vi "Autonomous Independent.vi"   [LabVIEW 2020]
doc: "This VI is called when autonomous begins, and will automatically be terminated when autonomous ends. You can carry out timed or sensor driven robot movement independently without needing to return to the caller."
uses:
  <vilib>/Rock Robotics/WPI/ThirdParty/Phoenix-LabVIEW/Motor Controller/Controls/CTRE_Phoenix_MotorControl_ControlMode.ctl
  <vilib>/Rock Robotics/WPI/Solenoid/WPI_SolenoidValue.ctl
  <vilib>/Rock Robotics/WPI/Utilities/WPI_GetSetVariantRefNum.vi
  <vilib>/Rock Robotics/Network Tables/NT Read String.vi
  <vilib>/Rock Robotics/Network Tables/NT Write Numeric Array.vi
  <vilib>/Rock Robotics/WPI/Solenoid/WPI_SolenoidSetEnum.vi
panel:
  # "Be sure to right-click and choose Data Operations>>Make Current Value default if you want to save the array values with the VI"
types:
  T1 = typedef "WPI_JoystickDevRef.ctl" = cluster{"Device":T2}
  T2 = typedef "WPI_JoystickDeviceEnum.ctl" = enum16{"USB 0", "USB 1", "USB 2", "USB 3", "USB 4", "USB 5"}
  T3 = typedef "WPI_MotorControlDeviceRef.ctl" = cluster{"DeviceStatus":errorcluster, "Type":T4, "PWM":cluster{"PWM Channel":T5, "DeadBand":T6}, "CAN":cluster{"Device Number":u8, "SetOutput VI Ref":variant, "GetOutput VI Ref":variant, "Enable VI Ref":variant, "Disable VI Ref":variant, "Data":variant}, "Invert":bool, "DIO PWM":cluster{"PWM \"Enable\" Channel":T5, "DIOChannel":T7, "PWM Rate":dbl}}
  T4 = typedef "WPI_MotorControlType.ctl" = enum16{"PWM", "CAN", "DIO PWM"}
  T5 = typedef "FPGA_DIOPWMChannel.ctl" = enum8{"PWM 0", "PWM 1", "PWM 2", "PWM 3", "PWM 4", "PWM 5", "PWM 6", "PWM 7", "PWM 8", "PWM 9", "PWM MXP 0", "PWM MXP 1", "PWM MXP 2", "PWM MXP 3", "PWM MXP 4", "PWM MXP 5", "PWM MXP 6", "PWM MXP 7", "PWM MXP 8", "PWM MXP 9", "Invalid"}
  T6 = typedef "WPI_PWMDeadband.ctl" = cluster{"Name":string, "maxPositivePwm":i32, "minPositivePwm":i32, "centerPwm":i32, "maxNegativePwm":i32, "minNegativePwm":i32, "angularRange":u16}
  T7 = typedef "FPGA_DIOChannel.ctl" = enum8{"DIO 0", "DIO 1", "DIO 2", "DIO 3", "DIO 4", "DIO 5", "DIO 6", "DIO 7", "DIO 8", "DIO 9", "DIO MXP 0", "DIO MXP 1", "DIO MXP 2", "DIO MXP 3", "DIO MXP 4", "DIO MXP 5", "DIO MXP 6", "DIO MXP 7", "DIO MXP 8", "DIO MXP 9", "DIO MXP 10", "DIO MXP 11", "DIO MXP 12", "DIO MXP 13", "DIO MXP 14", "DIO MXP 15", "SPI Port CS1", "SPI Port CS2", "SPI Port CS3", "SPI Port MISO", "SPI Port MOSI", "Invalid"}
  T8 = typedef "WPI_RobotDriveDevRef.ctl" = cluster{"DevStatus":errorcluster, "Motors[]":T3[], "Square Inputs":bool, "Max Output":dbl}
  T9 = typedef "WPI_SolenoidDevRef.ctl" = cluster{"DevStatus":errorcluster, "Pneumatics Control Module":u8, "Forward Solenoid Channel":T10, "Reverse Solenoid Channel":T10}
  T10 = typedef "WPI_SolenoidChannel.ctl" = enum8{"Solenoid 0", "Solenoid 1", "Solenoid 2", "Solenoid 3", "Solenoid 4", "Solenoid 5", "Solenoid 6", "Solenoid 7", "Solenoid 8", "Solenoid 9", "Solenoid 10", "Solenoid 11", "Solenoid 12", "Solenoid 13", "Solenoid 14", "Solenoid 15", "Invalid"}
  T11 = typedef "WPI_DigitalInputDevRef.ctl" = cluster{"DevStatus":errorcluster, "DIO Channel":T7}
  T12 = typedef "WPI_SolenoidValue.ctl" = enum16{"Off", "On", "Forward", "Reverse"}
  T13 = typedef "CTRE_Phoenix_MotorControl_ControlMode.ctl" = u16
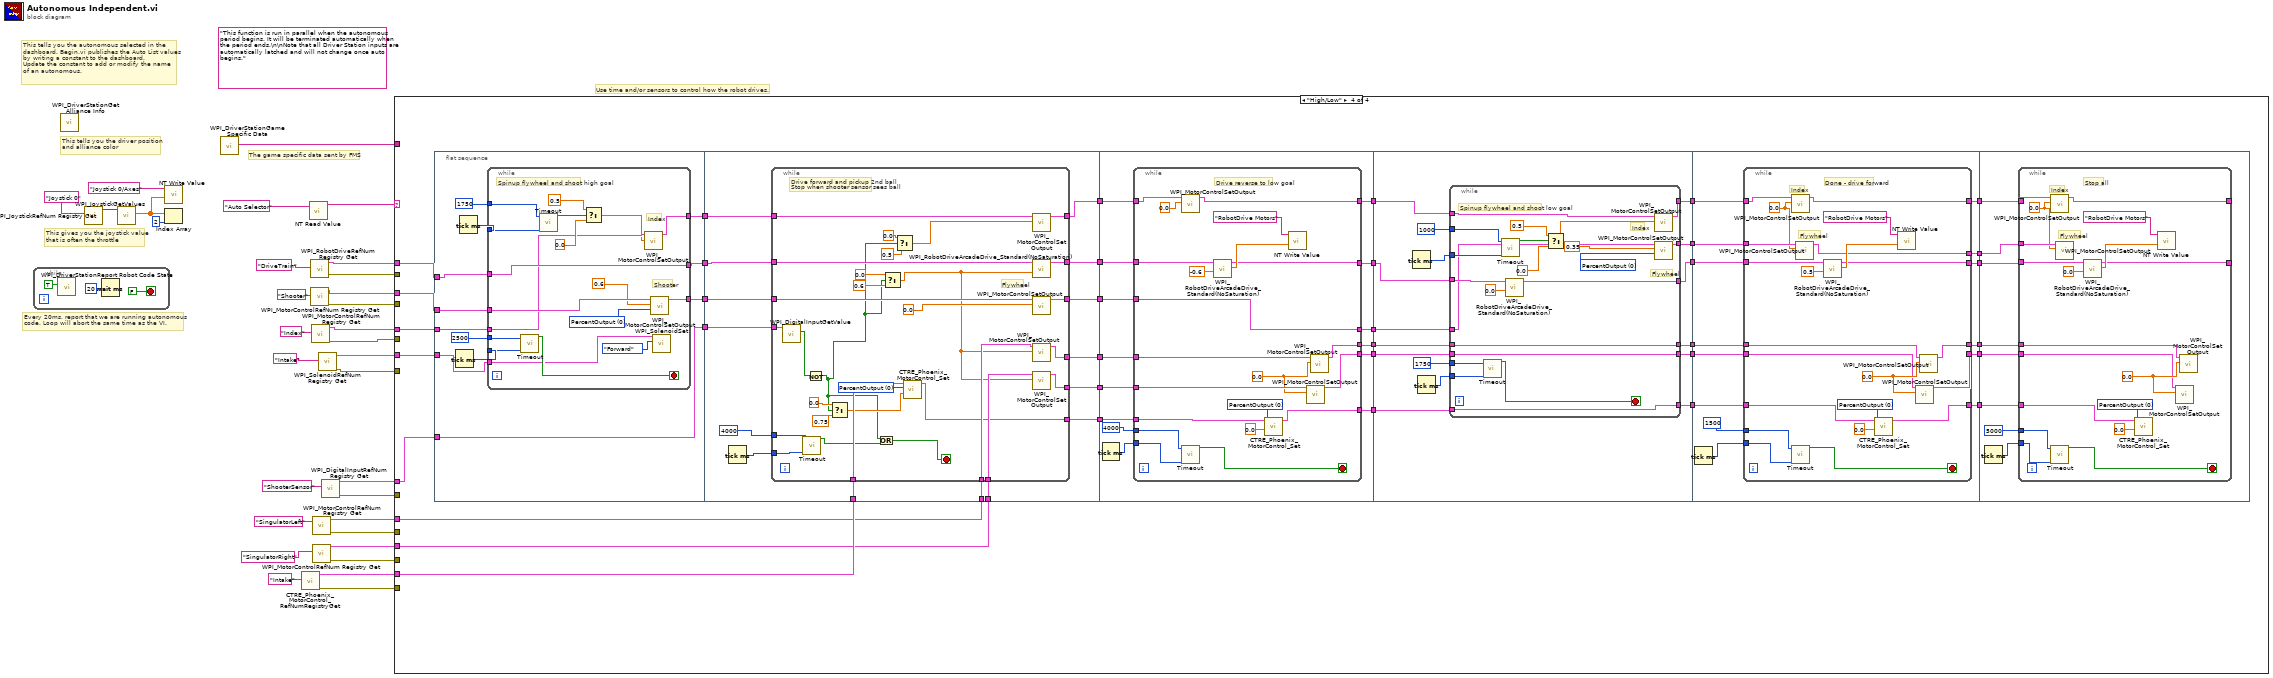
[diagram p0: block diagram]
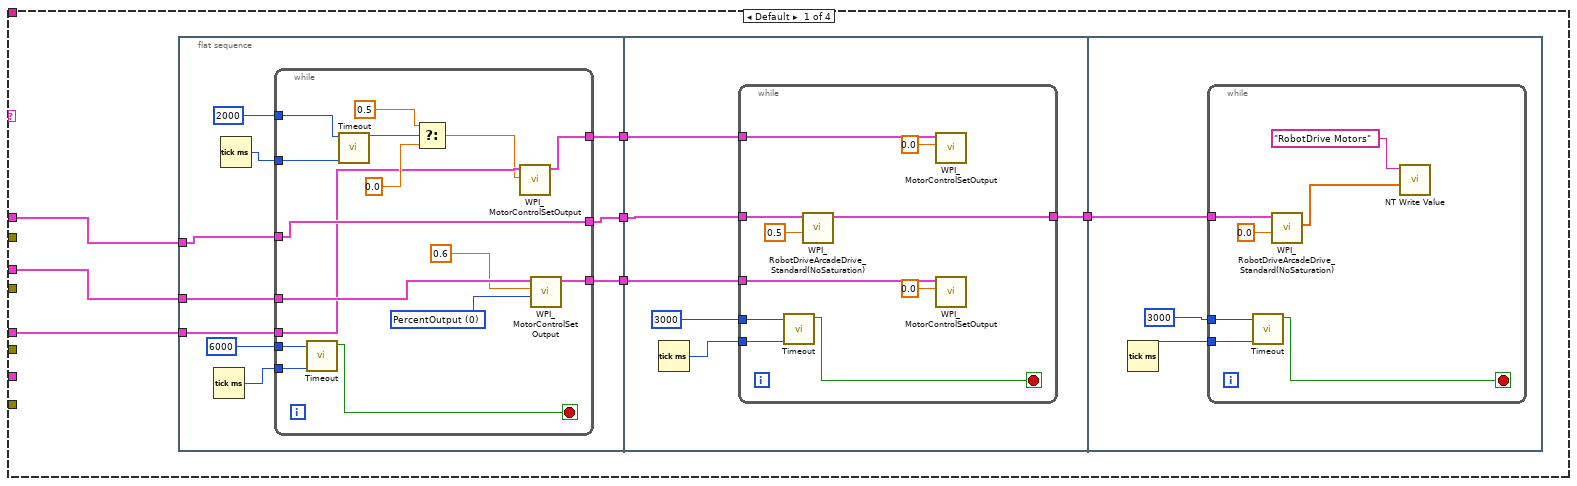
[diagram p2: hidden frame]
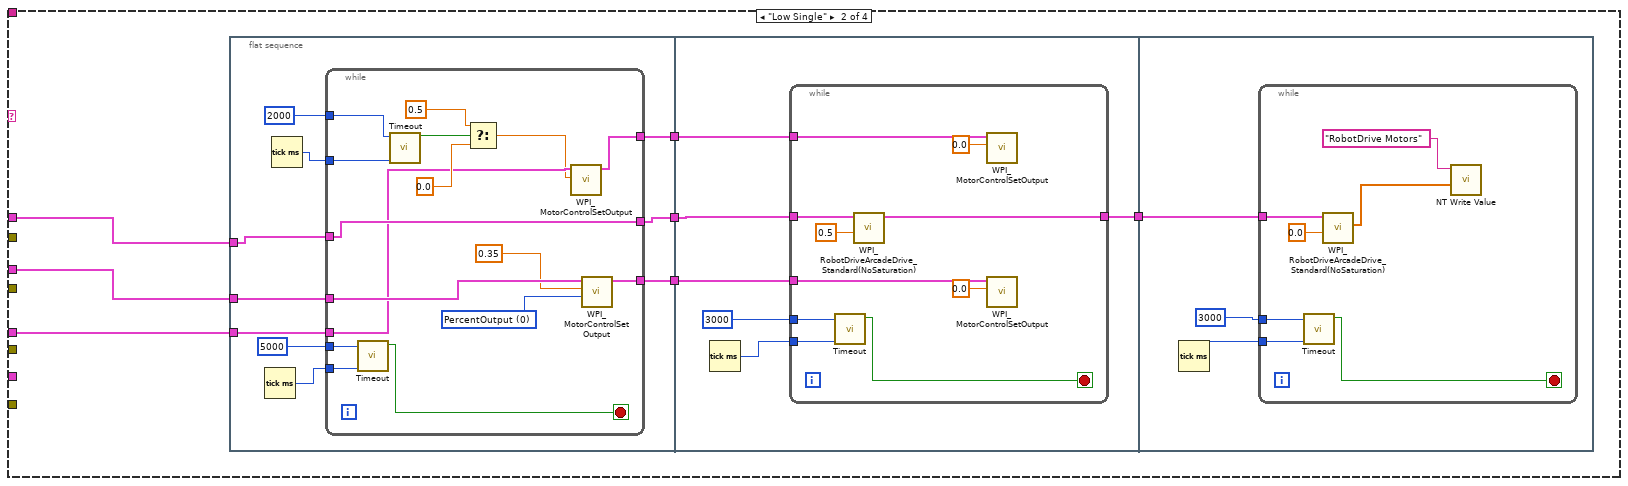
[diagram p3: hidden frame]
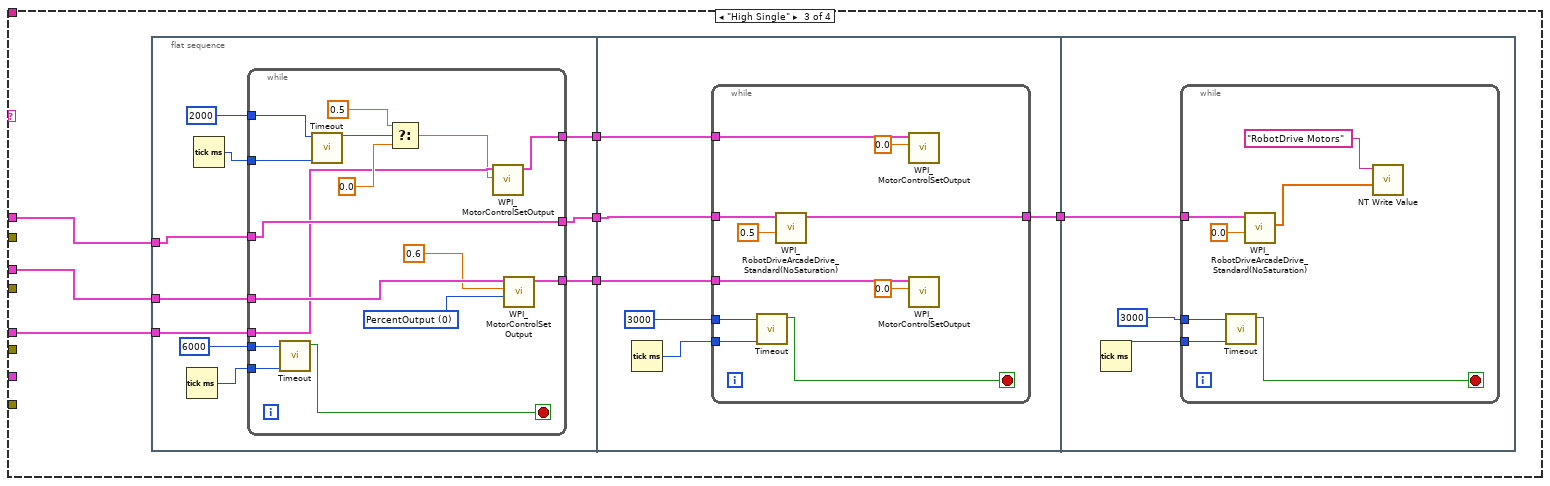
[diagram p4: hidden frame]
diagram:
  (unwired) "This function is run in parallel when the autonomous period begins. It will be terminated automatically when the period ends.\n\nNote that all Driver Station inputs are automatically latched and will not change once auto begins."
  # "The game specific data sent by FMS"
  # "This tells you the autonomous selected in the \ndashboard. Begin.vi publishes the Auto List values\nby writing a constant to the dashboard.\nUpdate the constant to add or modify the name\nof an autonomous."
  # "Every 20ms, report that we are running autonomous\ncode. Loop will abort the same time as the VI."
  # "This gives you the joystick value\nthat is often the throttle"
  # "Use time and/or sensors to control how the robot drives."
  # "This tells you the driver position\nand alliance color"
  n1 = while {
    stop <- FALSE stop-if-true
    n2 = call <vilib>:"WPI_DriverStationReport Robot Code State.vi"("Autonomous"=TRUE) -> ()  [unwired: 10 in, 1 out]
    n3 = Wait (ms)(milliseconds to wait=u32 20) -> ()  [unwired: 1 out]
  }
  n4 = call <vilib>:"WPI_DriverStationGet Alliance Info.vi"() -> ()  [unwired: 12 out]
  n5 = call <vilib>:"WPI_JoystickRefNum Registry Get.vi"("refnum name"="Joystick 0") -> ("JoystickDevRef"=w31:T1)  [unwired: 1 in, 9 out]
  n6 = call <vilib>:"WPI_JoystickGetValues.vi"("JoystickDevRef"=w31) -> ("Axes"=w27:dbl[])  [unwired: 6 in, 4 out]
  n7 = call-poly <vilib>:"NT Write Value.vi"("Numeric Array"=w27, "Name"="Joystick 0/Axes") -> ()  [unwired: 9 in, 1 out]
  n8 = Index Array(array=w27, index=2) -> ()  [unwired: 1 out]
  n9 = call <vilib>:"WPI_DriverStationGame Specific Data.vi"() -> ("Game Specific Data"=w25:string)  [unwired: 11 in]
  n10 = call <vilib>:"CTRE_Phoenix_MotorControl_RefNumRegistryGet.vi"("refnum name"="Intake") -> ("error out"=w2:errorcluster, "PhoenixMotorControlDevRef"=w3:T3)  [unwired: 9 in]
  n11 = call-poly <vilib>:"NT Read Value.vi"("Name"="Auto Selector") -> ("String"=w28:string)  [unwired: 9 in, 1 out]
  n12 = call <vilib>:"WPI_RobotDriveRefNum Registry Get.vi"("refnum name"="DriveTrain") -> ("error out"=w13:errorcluster, "RobotDriveDevRef"=w23:T8)  [unwired: 9 in]
  n13 = call <vilib>:"WPI_MotorControlRefNum Registry Get.vi"("refnum name"="Shooter") -> ("error out"=w14:errorcluster, "MotorControlDevRef"=w21:T3)  [unwired: 9 in]
  n14 = call <vilib>:"WPI_MotorControlRefNum Registry Get.vi"("refnum name"="Index") -> ("error out"=w15:errorcluster, "MotorControlDevRef"=w19:T3)  [unwired: 9 in]
  n15 = call <vilib>:"WPI_MotorControlRefNum Registry Get.vi"("refnum name"="SingulatorRight") -> ("error out"=w4:errorcluster, "MotorControlDevRef"=w7:T3)  [unwired: 9 in]
  n16 = call <vilib>:"WPI_MotorControlRefNum Registry Get.vi"("refnum name"="SingulatorLeft") -> ("error out"=w5:errorcluster, "MotorControlDevRef"=w8:T3)  [unwired: 9 in]
  n17 = call <vilib>:"WPI_SolenoidRefNum Registry Get.vi"("refnum name"="Intake") -> ("error out"=w16:errorcluster, "SolenoidDevRef"=w1:T9)  [unwired: 9 in]
  n18 = call <vilib>:"WPI_DigitalInputRefNum Registry Get.vi"("refnum name"="ShooterSensor") -> ("error out"=w11:errorcluster, "DigitalInputDevRef"=w12:T11)  [unwired: 9 in]
  n19 = case shown="\"High/Low\"" w28 {
    tunnel: w25 -> [_ _ _ _]
    tunnel: w23 -> [w42 w97 w156 w244]
    tunnel: w21 -> [w40 w96 w155 w243]
    tunnel: w19 -> [w38 w95 w154 w242]
    tunnel: w16 -> [_ _ _ _]
    tunnel: w15 -> [_ _ _ _]
    tunnel: w14 -> [_ _ _ _]
    tunnel: w13 -> [_ _ _ _]
    tunnel: w12 -> [_ _ _ w240]
    tunnel: w11 -> [_ _ _ _]
    tunnel: w8 -> [_ _ _ w233]
    tunnel: w7 -> [_ _ _ w232]
    tunnel: w5 -> [_ _ _ _]
    tunnel: w4 -> [_ _ _ _]
    tunnel: w3 -> [_ _ _ w241]
    tunnel: w2 -> [_ _ _ _]
    tunnel: w1 -> [_ _ _ w228]
    frame Default {
      n20 = flat-sequence {
        tunnel: w42 -> [w49]
        tunnel: [w48] -> w41
        tunnel: w40 -> [w52]
        tunnel: w38 -> [w45]
        tunnel: [w44] -> w37
        tunnel: [w43] -> w36
        tunnel: w41 -> [w74]
        tunnel: [w71] -> w39
        tunnel: w37 -> [w70]
        tunnel: w36 -> [w69]
        tunnel: w39 -> [w87]
        frame #0 {
          n21 = Tick Count (ms)() -> (millisecond timer value=w50:u32)
          n22 = Tick Count (ms)() -> (millisecond timer value=w46:u32)
          n23 = while {
            tunnel: w52 -> [w67]
            tunnel: 6000 -> [w66]
            tunnel: w50 -> [w65]
            tunnel: w49 -> [w63]
            tunnel: [w63] -> w48
            tunnel: 2000 -> [w62]
            tunnel: w46 -> [w61]
            tunnel: w45 -> [w57]
            tunnel: [w54] -> w44
            tunnel: [w53] -> w43
            stop <- w64 stop-if-true
            w68 = T13 0 items=["PercentOutput"=0, "Position"=1, "Velocity"=2, "Current"=3, "Follower"=5, "MotionProfile"=6, "MotionMagic"=7, "MotionProfileArc"=10, "Disabled"=15] ("Control Mode")
            n24 = call "Timeout.vi"("Start Time In"=w65, "Limit In"=w66) -> ("Timeout"=w64:bool)  [unwired: 8 in, 1 out]
            n25 = call "Timeout.vi"("Start Time In"=w61, "Limit In"=w62) -> ("Timeout"=w60:bool)  [unwired: 8 in, 1 out]
            n26 = Select(t=0.5 ("Output"), s=w60, f=0.0) -> (s? t:f=w55:dbl)
            n27 = call <vilib>:"WPI_MotorControlSetOutput.vi"("Output"=w55, "MotorControlDevRef"=w57) -> ("MotorControlDevRef"=w54:T3)  [unwired: 7 in, 2 out]
            n28 = call <vilib>:"WPI_MotorControlSetOutput.vi"("options"=w68, "Output"=0.6, "MotorControlDevRef"=w67) -> ("MotorControlDevRef"=w53:T3)  [unwired: 6 in, 2 out]
          }
        }
        frame #1 {
          n29 = Tick Count (ms)() -> (millisecond timer value=w73:u32)
          n30 = while {
            tunnel: w74 -> [w84]
            tunnel: w73 -> [w83]
            tunnel: 3000 -> [w82]
            tunnel: [w79] -> w71
            tunnel: w70 -> [w78]
            tunnel: w69 -> [w77]
            stop <- w81 stop-if-true
            n31 = call "Timeout.vi"("Start Time In"=w83, "Limit In"=w82) -> ("Timeout"=w81:bool)  [unwired: 8 in, 1 out]
            n32 = call <vilib>:"WPI_RobotDriveArcadeDrive_Standard(NoSaturation).vi"("Y axis value"=0.5, "RobotDriveDevRef"=w84) -> ("RobotDriveDevRef"=w79:T8)  [unwired: 2 in, 7 out]
            n33 = call <vilib>:"WPI_MotorControlSetOutput.vi"("Output"=0.0, "MotorControlDevRef"=w78) -> ()  [unwired: 7 in, 3 out]
            n34 = call <vilib>:"WPI_MotorControlSetOutput.vi"("Output"=0.0, "MotorControlDevRef"=w77) -> ()  [unwired: 7 in, 3 out]
          }
        }
        frame #2 {
          n35 = Tick Count (ms)() -> (millisecond timer value=w85:u32)
          n36 = while {
            tunnel: w87 -> [w92]
            tunnel: w85 -> [w91]
            tunnel: 3000 -> [w90]
            stop <- w89 stop-if-true
            n37 = call "Timeout.vi"("Start Time In"=w91, "Limit In"=w90) -> ("Timeout"=w89:bool)  [unwired: 8 in, 1 out]
            n38 = call <vilib>:"WPI_RobotDriveArcadeDrive_Standard(NoSaturation).vi"("Y axis value"=0.0, "RobotDriveDevRef"=w92) -> ("Motor Values"=w94:dbl[])  [unwired: 2 in, 7 out]
            n39 = call-poly <vilib>:"NT Write Value.vi"("Numeric Array"=w94, "Name"="RobotDrive Motors") -> ()  [unwired: 9 in, 1 out]
          }
        }
      }
    }
    frame "Low Single" {
      n40 = flat-sequence {
        tunnel: w97 -> [w108]
        tunnel: [w107] -> w101
        tunnel: w96 -> [w111]
        tunnel: w95 -> [w104]
        tunnel: [w103] -> w100
        tunnel: [w102] -> w99
        tunnel: w101 -> [w133]
        tunnel: [w130] -> w98
        tunnel: w100 -> [w129]
        tunnel: w99 -> [w128]
        tunnel: w98 -> [w146]
        frame #0 {
          n41 = Tick Count (ms)() -> (millisecond timer value=w109:u32)
          n42 = Tick Count (ms)() -> (millisecond timer value=w105:u32)
          n43 = while {
            tunnel: w111 -> [w126]
            tunnel: 5000 -> [w125]
            tunnel: w109 -> [w124]
            tunnel: w108 -> [w122]
            tunnel: [w122] -> w107
            tunnel: 2000 -> [w121]
            tunnel: w105 -> [w120]
            tunnel: w104 -> [w116]
            tunnel: [w113] -> w103
            tunnel: [w112] -> w102
            stop <- w123 stop-if-true
            w127 = T13 0 items=["PercentOutput"=0, "Position"=1, "Velocity"=2, "Current"=3, "Follower"=5, "MotionProfile"=6, "MotionMagic"=7, "MotionProfileArc"=10, "Disabled"=15] ("Control Mode")
            n44 = call "Timeout.vi"("Start Time In"=w124, "Limit In"=w125) -> ("Timeout"=w123:bool)  [unwired: 8 in, 1 out]
            n45 = call "Timeout.vi"("Start Time In"=w120, "Limit In"=w121) -> ("Timeout"=w119:bool)  [unwired: 8 in, 1 out]
            n46 = Select(t=0.5 ("Output"), s=w119, f=0.0) -> (s? t:f=w114:dbl)
            n47 = call <vilib>:"WPI_MotorControlSetOutput.vi"("Output"=w114, "MotorControlDevRef"=w116) -> ("MotorControlDevRef"=w113:T3)  [unwired: 7 in, 2 out]
            n48 = call <vilib>:"WPI_MotorControlSetOutput.vi"("options"=w127, "Output"=0.35, "MotorControlDevRef"=w126) -> ("MotorControlDevRef"=w112:T3)  [unwired: 6 in, 2 out]
          }
        }
        frame #1 {
          n49 = Tick Count (ms)() -> (millisecond timer value=w132:u32)
          n50 = while {
            tunnel: w133 -> [w143]
            tunnel: w132 -> [w142]
            tunnel: 3000 -> [w141]
            tunnel: [w138] -> w130
            tunnel: w129 -> [w137]
            tunnel: w128 -> [w136]
            stop <- w140 stop-if-true
            n51 = call "Timeout.vi"("Start Time In"=w142, "Limit In"=w141) -> ("Timeout"=w140:bool)  [unwired: 8 in, 1 out]
            n52 = call <vilib>:"WPI_RobotDriveArcadeDrive_Standard(NoSaturation).vi"("Y axis value"=0.5, "RobotDriveDevRef"=w143) -> ("RobotDriveDevRef"=w138:T8)  [unwired: 2 in, 7 out]
            n53 = call <vilib>:"WPI_MotorControlSetOutput.vi"("Output"=0.0, "MotorControlDevRef"=w137) -> ()  [unwired: 7 in, 3 out]
            n54 = call <vilib>:"WPI_MotorControlSetOutput.vi"("Output"=0.0, "MotorControlDevRef"=w136) -> ()  [unwired: 7 in, 3 out]
          }
        }
        frame #2 {
          n55 = Tick Count (ms)() -> (millisecond timer value=w144:u32)
          n56 = while {
            tunnel: w146 -> [w151]
            tunnel: w144 -> [w150]
            tunnel: 3000 -> [w149]
            stop <- w148 stop-if-true
            n57 = call "Timeout.vi"("Start Time In"=w150, "Limit In"=w149) -> ("Timeout"=w148:bool)  [unwired: 8 in, 1 out]
            n58 = call <vilib>:"WPI_RobotDriveArcadeDrive_Standard(NoSaturation).vi"("Y axis value"=0.0, "RobotDriveDevRef"=w151) -> ("Motor Values"=w153:dbl[])  [unwired: 2 in, 7 out]
            n59 = call-poly <vilib>:"NT Write Value.vi"("Numeric Array"=w153, "Name"="RobotDrive Motors") -> ()  [unwired: 9 in, 1 out]
          }
        }
      }
    }
    frame "High Single" {
      n60 = flat-sequence {
        tunnel: w156 -> [w167]
        tunnel: [w166] -> w160
        tunnel: w155 -> [w170]
        tunnel: w154 -> [w163]
        tunnel: [w162] -> w159
        tunnel: [w161] -> w158
        tunnel: w160 -> [w192]
        tunnel: [w189] -> w157
        tunnel: w159 -> [w188]
        tunnel: w158 -> [w187]
        tunnel: w157 -> [w205]
        frame #0 {
          n61 = Tick Count (ms)() -> (millisecond timer value=w168:u32)
          n62 = Tick Count (ms)() -> (millisecond timer value=w164:u32)
          n63 = while {
            tunnel: w170 -> [w185]
            tunnel: 6000 -> [w184]
            tunnel: w168 -> [w183]
            tunnel: w167 -> [w181]
            tunnel: [w181] -> w166
            tunnel: 2000 -> [w180]
            tunnel: w164 -> [w179]
            tunnel: w163 -> [w175]
            tunnel: [w172] -> w162
            tunnel: [w171] -> w161
            stop <- w182 stop-if-true
            w186 = T13 0 items=["PercentOutput"=0, "Position"=1, "Velocity"=2, "Current"=3, "Follower"=5, "MotionProfile"=6, "MotionMagic"=7, "MotionProfileArc"=10, "Disabled"=15] ("Control Mode")
            n64 = call "Timeout.vi"("Start Time In"=w183, "Limit In"=w184) -> ("Timeout"=w182:bool)  [unwired: 8 in, 1 out]
            n65 = call "Timeout.vi"("Start Time In"=w179, "Limit In"=w180) -> ("Timeout"=w178:bool)  [unwired: 8 in, 1 out]
            n66 = Select(t=0.5 ("Output"), s=w178, f=0.0) -> (s? t:f=w173:dbl)
            n67 = call <vilib>:"WPI_MotorControlSetOutput.vi"("Output"=w173, "MotorControlDevRef"=w175) -> ("MotorControlDevRef"=w172:T3)  [unwired: 7 in, 2 out]
            n68 = call <vilib>:"WPI_MotorControlSetOutput.vi"("options"=w186, "Output"=0.6, "MotorControlDevRef"=w185) -> ("MotorControlDevRef"=w171:T3)  [unwired: 6 in, 2 out]
          }
        }
        frame #1 {
          n69 = Tick Count (ms)() -> (millisecond timer value=w191:u32)
          n70 = while {
            tunnel: w192 -> [w202]
            tunnel: w191 -> [w201]
            tunnel: 3000 -> [w200]
            tunnel: [w197] -> w189
            tunnel: w188 -> [w196]
            tunnel: w187 -> [w195]
            stop <- w199 stop-if-true
            n71 = call "Timeout.vi"("Start Time In"=w201, "Limit In"=w200) -> ("Timeout"=w199:bool)  [unwired: 8 in, 1 out]
            n72 = call <vilib>:"WPI_RobotDriveArcadeDrive_Standard(NoSaturation).vi"("Y axis value"=0.5, "RobotDriveDevRef"=w202) -> ("RobotDriveDevRef"=w197:T8)  [unwired: 2 in, 7 out]
            n73 = call <vilib>:"WPI_MotorControlSetOutput.vi"("Output"=0.0, "MotorControlDevRef"=w196) -> ()  [unwired: 7 in, 3 out]
            n74 = call <vilib>:"WPI_MotorControlSetOutput.vi"("Output"=0.0, "MotorControlDevRef"=w195) -> ()  [unwired: 7 in, 3 out]
          }
        }
        frame #2 {
          n75 = Tick Count (ms)() -> (millisecond timer value=w203:u32)
          n76 = while {
            tunnel: w205 -> [w210]
            tunnel: w203 -> [w209]
            tunnel: 3000 -> [w208]
            stop <- w207 stop-if-true
            n77 = call "Timeout.vi"("Start Time In"=w209, "Limit In"=w208) -> ("Timeout"=w207:bool)  [unwired: 8 in, 1 out]
            n78 = call <vilib>:"WPI_RobotDriveArcadeDrive_Standard(NoSaturation).vi"("Y axis value"=0.0, "RobotDriveDevRef"=w210) -> ("Motor Values"=w212:dbl[])  [unwired: 2 in, 7 out]
            n79 = call-poly <vilib>:"NT Write Value.vi"("Numeric Array"=w212, "Name"="RobotDrive Motors") -> ()  [unwired: 9 in, 1 out]
          }
        }
      }
    }
    frame "High/Low" {
      n80 = flat-sequence {
        tunnel: w244 -> [w257]
        tunnel: [w256] -> w248
        tunnel: w243 -> [w260]
        tunnel: w242 -> [w253]
        tunnel: [w252] -> w247
        tunnel: [w251] -> w246
        tunnel: w240 -> [w250]
        tunnel: [w250] -> w239
        tunnel: w228 -> [w249]
        tunnel: w248 -> [w293]
        tunnel: [w290] -> w245
        tunnel: w247 -> [w289]
        tunnel: w246 -> [w288]
        tunnel: w241 -> [w287]
        tunnel: w239 -> [w286]
        tunnel: [w285] -> w236
        tunnel: [w284] -> w234
        tunnel: w233 -> [w283]
        tunnel: w232 -> [w282]
        tunnel: [w281] -> w231
        tunnel: [w280] -> w230
        tunnel: [w279] -> w229
        tunnel: w245 -> [w337]
        tunnel: [w334] -> w238
        tunnel: [w333] -> w237
        tunnel: w236 -> [w332]
        tunnel: [w331] -> w235
        tunnel: w234 -> [w330]
        tunnel: w231 -> [w329]
        tunnel: w230 -> [w328]
        tunnel: w229 -> [w327]
        tunnel: [w326] -> w223
        tunnel: [w325] -> w221
        tunnel: [w324] -> w219
        tunnel: w238 -> [w370]
        tunnel: w237 -> [w369]
        tunnel: w235 -> [w368]
        tunnel: [w367] -> w227
        tunnel: [w366] -> w226
        tunnel: [w365] -> w225
        tunnel: [w364] -> w224
        tunnel: w223 -> [w363]
        tunnel: [w362] -> w222
        tunnel: w221 -> [w361]
        tunnel: [w360] -> w220
        tunnel: w219 -> [w359]
        tunnel: w227 -> [w407]
        tunnel: w226 -> [w406]
        tunnel: w225 -> [w405]
        tunnel: w224 -> [w404]
        tunnel: w222 -> [w403]
        tunnel: w220 -> [w402]
        tunnel: [w401] -> w218
        tunnel: [w400] -> w217
        tunnel: [w399] -> w216
        tunnel: [w398] -> w215
        tunnel: [w397] -> w214
        tunnel: [w396] -> w213
        tunnel: w218 -> [w439]
        tunnel: w217 -> [w438]
        tunnel: w216 -> [w437]
        tunnel: w215 -> [w436]
        tunnel: w214 -> [w435]
        tunnel: w213 -> [w434]
        frame #0 {
          n81 = Tick Count (ms)() -> (millisecond timer value=w258:u32)
          n82 = Tick Count (ms)() -> (millisecond timer value=w254:u32)
          n83 = while {
            tunnel: w260 -> [w277]
            tunnel: 2500 -> [w276]
            tunnel: w258 -> [w275]
            tunnel: w257 -> [w273]
            tunnel: [w273] -> w256
            tunnel: 1750 -> [w272]
            tunnel: w254 -> [w271]
            tunnel: w253 -> [w267]
            tunnel: [w264] -> w252
            tunnel: [w263] -> w251
            tunnel: w249 -> [w261]
            stop <- w274 stop-if-true
            w278 = T13 0 items=["PercentOutput"=0, "Position"=1, "Velocity"=2, "Current"=3, "Follower"=5, "MotionProfile"=6, "MotionMagic"=7, "MotionProfileArc"=10, "Disabled"=15] ("Control Mode")
            # "Shooter"
            # "Index"
            # "Spinup flywheel and shoot high goal"
            n84 = call "Timeout.vi"("Start Time In"=w275, "Limit In"=w276) -> ("Timeout"=w274:bool)  [unwired: 8 in, 1 out]
            n85 = call "Timeout.vi"("Start Time In"=w271, "Limit In"=w272) -> ("Timeout"=w270:bool)  [unwired: 8 in, 1 out]
            n86 = Select(t=0.5 ("Output"), s=w270, f=0.0) -> (s? t:f=w265:dbl)
            n87 = call <vilib>:"WPI_MotorControlSetOutput.vi"("Output"=w265, "MotorControlDevRef"=w267) -> ("MotorControlDevRef"=w264:T3)  [unwired: 7 in, 2 out]
            n88 = call <vilib>:"WPI_MotorControlSetOutput.vi"("options"=w278, "Output"=0.6, "MotorControlDevRef"=w277) -> ("MotorControlDevRef"=w263:T3)  [unwired: 6 in, 2 out]
            n89 = call-poly <vilib>:"WPI_SolenoidSet.vi"("Value"=WPI_SolenoidValue."Forward", "SolenoidDevRef"=w261) -> ()  [unwired: 8 in, 2 out]
          }
        }
        frame #1 {
          n90 = Tick Count (ms)() -> (millisecond timer value=w292:u32)
          n91 = while {
            tunnel: w293 -> [w323]
            tunnel: w292 -> [w322]
            tunnel: 4000 -> [w321]
            tunnel: [w320] -> w290
            tunnel: w289 -> [w319]
            tunnel: w288 -> [w318]
            tunnel: w287 -> [w314]
            tunnel: w286 -> [w309]
            tunnel: [w301] -> w285
            tunnel: [w300] -> w284
            tunnel: w283 -> [w299]
            tunnel: w282 -> [w298]
            tunnel: [w296] -> w281
            tunnel: [w295] -> w280
            tunnel: [w294] -> w279
            stop <- w304 stop-if-true
            w313 = T13 0 items=["PercentOutput"=0, "Position"=1, "Velocity"=2, "Current"=3, "Follower"=5, "MotionProfile"=6, "MotionMagic"=7, "MotionProfileArc"=10, "Disabled"=15] ("Control Mode")
            # "Flywheel"
            # "Drive forward and pickup 2nd ball\nStop when shooter sensor sees ball"
            n92 = call <vilib>:"WPI_DigitalInputGetValue.vi"("DigitalInputDevRef"=w309) -> ("Value"=w308:bool)  [unwired: 8 in, 2 out]
            n93 = call "Timeout.vi"("Start Time In"=w322, "Limit In"=w321) -> ("Timeout"=w303:bool)  [unwired: 8 in, 1 out]
            n94 = Not(x=w308) -> (.not. x?=w302:bool)
            n95 = Select(t=0.0 ("Output"), s=w302, f=0.75) -> (s? t:f=w312:dbl)
            n96 = Or(x=w302, y=w303) -> (x .or. y?=w304:bool)
            n97 = Select(t=0.0, s=w302, f=0.6) -> (s? t:f=w297:dbl)
            n98 = Select(t=0.0, s=w302, f=0.5 ("Output")) -> (s? t:f=w316:dbl)
            n99 = call <vilib>:"CTRE_Phoenix_MotorControl_Set.vi"("Output"=w312, "Control Mode"=w313, "PhoenixMotorControlDevRef"=w314) -> ("PhoenixMotorControlDevRef"=w294:T3)  [unwired: 7 in, 1 out]
            n100 = call <vilib>:"WPI_MotorControlSetOutput.vi"("Output"=w316, "MotorControlDevRef"=w319) -> ("MotorControlDevRef"=w300:T3)  [unwired: 7 in, 2 out]
            n101 = call <vilib>:"WPI_RobotDriveArcadeDrive_Standard(NoSaturation).vi"("Y axis value"=w297, "RobotDriveDevRef"=w323) -> ("RobotDriveDevRef"=w320:T8)  [unwired: 2 in, 7 out]
            n102 = call <vilib>:"WPI_MotorControlSetOutput.vi"("Output"=0.0, "MotorControlDevRef"=w318) -> ("MotorControlDevRef"=w301:T3)  [unwired: 7 in, 2 out]
            n103 = call <vilib>:"WPI_MotorControlSetOutput.vi"("Output"=w297, "MotorControlDevRef"=w299) -> ("MotorControlDevRef"=w296:T3)  [unwired: 7 in, 2 out]
            n104 = call <vilib>:"WPI_MotorControlSetOutput.vi"("Output"=w297, "MotorControlDevRef"=w298) -> ("MotorControlDevRef"=w295:T3)  [unwired: 7 in, 2 out]
          }
        }
        frame #2 {
          n105 = Tick Count (ms)() -> (millisecond timer value=w335:u32)
          n106 = while {
            tunnel: w337 -> [w356]
            tunnel: w335 -> [w355]
            tunnel: 4000 -> [w354]
            tunnel: [w351] -> w334
            tunnel: [w350] -> w333
            tunnel: w332 -> [w350]
            tunnel: [w346] -> w331
            tunnel: w330 -> [w347]
            tunnel: w329 -> [w349]
            tunnel: w328 -> [w348]
            tunnel: w327 -> [w343]
            tunnel: [w340] -> w326
            tunnel: [w339] -> w325
            tunnel: [w338] -> w324
            stop <- w353 stop-if-true
            w341 = T13 0 items=["PercentOutput"=0, "Position"=1, "Velocity"=2, "Current"=3, "Follower"=5, "MotionProfile"=6, "MotionMagic"=7, "MotionProfileArc"=10, "Disabled"=15] ("Control Mode")
            w345 = 0.0 ("Output")
            # "Drive reverse to low goal"
            n107 = call <vilib>:"WPI_MotorControlSetOutput.vi"("Output"=0.0, "MotorControlDevRef"=w347) -> ("MotorControlDevRef"=w346:T3)  [unwired: 7 in, 2 out]
            n108 = call "Timeout.vi"("Start Time In"=w355, "Limit In"=w354) -> ("Timeout"=w353:bool)  [unwired: 8 in, 1 out]
            n109 = call <vilib>:"WPI_RobotDriveArcadeDrive_Standard(NoSaturation).vi"("Y axis value"=-0.6, "RobotDriveDevRef"=w356) -> ("Motor Values"=w358:dbl[], "RobotDriveDevRef"=w351:T8)  [unwired: 2 in, 6 out]
            n110 = call <vilib>:"CTRE_Phoenix_MotorControl_Set.vi"("Output"=0.0, "Control Mode"=w341, "PhoenixMotorControlDevRef"=w343) -> ("PhoenixMotorControlDevRef"=w338:T3)  [unwired: 7 in, 1 out]
            n111 = call-poly <vilib>:"NT Write Value.vi"("Numeric Array"=w358, "Name"="RobotDrive Motors") -> ()  [unwired: 9 in, 1 out]
            n112 = call <vilib>:"WPI_MotorControlSetOutput.vi"("Output"=w345, "MotorControlDevRef"=w348) -> ("MotorControlDevRef"=w339:T3)  [unwired: 7 in, 2 out]
            n113 = call <vilib>:"WPI_MotorControlSetOutput.vi"("Output"=w345, "MotorControlDevRef"=w349) -> ("MotorControlDevRef"=w340:T3)  [unwired: 7 in, 2 out]
          }
        }
        frame #3 {
          n114 = Tick Count (ms)() -> (millisecond timer value=w371:u32)
          n115 = Tick Count (ms)() -> (millisecond timer value=w373:u32)
          n116 = while {
            tunnel: 1750 -> [w394]
            tunnel: w373 -> [w393]
            tunnel: 1000 -> [w391]
            tunnel: w371 -> [w390]
            tunnel: w370 -> [w384]
            tunnel: w369 -> [w383]
            tunnel: w368 -> [w381]
            tunnel: [w380] -> w367
            tunnel: [w379] -> w366
            tunnel: [w378] -> w365
            tunnel: [w377] -> w364
            tunnel: w363 -> [w377]
            tunnel: [w376] -> w362
            tunnel: w361 -> [w376]
            tunnel: [w375] -> w360
            tunnel: w359 -> [w375]
            stop <- w392 stop-if-true
            w395 = T13 0 items=["PercentOutput"=0, "Position"=1, "Velocity"=2, "Current"=3, "Follower"=5, "MotionProfile"=6, "MotionMagic"=7, "MotionProfileArc"=10, "Disabled"=15] ("Control Mode")
            # "Flywheel"
            # "Index"
            # "Spinup flywheel and shoot low goal"
            n117 = call "Timeout.vi"("Start Time In"=w393, "Limit In"=w394) -> ("Timeout"=w392:bool)  [unwired: 8 in, 1 out]
            n118 = call "Timeout.vi"("Start Time In"=w390, "Limit In"=w391) -> ("Timeout"=w389:bool)  [unwired: 8 in, 1 out]
            n119 = call <vilib>:"WPI_RobotDriveArcadeDrive_Standard(NoSaturation).vi"("Y axis value"=0.0, "RobotDriveDevRef"=w384) -> ("RobotDriveDevRef"=w379:T8)  [unwired: 2 in, 7 out]
            n120 = Select(t=0.5 ("Output"), s=w389, f=0.0) -> (s? t:f=w385:dbl)
            n121 = call <vilib>:"WPI_MotorControlSetOutput.vi"("Output"=w385, "MotorControlDevRef"=w381) -> ("MotorControlDevRef"=w380:T3)  [unwired: 7 in, 2 out]
            n122 = call <vilib>:"WPI_MotorControlSetOutput.vi"("options"=w395, "Output"=0.35, "MotorControlDevRef"=w383) -> ("MotorControlDevRef"=w378:T3)  [unwired: 6 in, 2 out]
          }
        }
        frame #4 {
          n123 = Tick Count (ms)() -> (millisecond timer value=w408:u32)
          n124 = while {
            tunnel: w408 -> [w429]
            tunnel: 1500 -> [w428]
            tunnel: [w425] -> w401
            tunnel: [w423] -> w399
            tunnel: w407 -> [w424]
            tunnel: w406 -> [w419]
            tunnel: w405 -> [w418]
            tunnel: w404 -> [w416]
            tunnel: w403 -> [w415]
            tunnel: w402 -> [w414]
            tunnel: [w413] -> w400
            tunnel: [w412] -> w398
            tunnel: [w411] -> w397
            tunnel: [w410] -> w396
            stop <- w427 stop-if-true
            w420 = T13 0 items=["PercentOutput"=0, "Position"=1, "Velocity"=2, "Current"=3, "Follower"=5, "MotionProfile"=6, "MotionMagic"=7, "MotionProfileArc"=10, "Disabled"=15] ("Control Mode")
            w417 = 0.0 ("Output")
            w422 = 0.0 ("Output")
            # "Index"
            # "Flywheel"
            # "Done - drive forward"
            n125 = call <vilib>:"WPI_MotorControlSetOutput.vi"("Output"=w417, "MotorControlDevRef"=w424) -> ("MotorControlDevRef"=w423:T3)  [unwired: 7 in, 2 out]
            n126 = call "Timeout.vi"("Start Time In"=w429, "Limit In"=w428) -> ("Timeout"=w427:bool)  [unwired: 8 in, 1 out]
            n127 = call <vilib>:"WPI_MotorControlSetOutput.vi"("Output"=w417, "MotorControlDevRef"=w418) -> ("MotorControlDevRef"=w413:T3)  [unwired: 7 in, 2 out]
            n128 = call <vilib>:"WPI_RobotDriveArcadeDrive_Standard(NoSaturation).vi"("Y axis value"=0.5, "RobotDriveDevRef"=w419) -> ("Motor Values"=w431:dbl[], "RobotDriveDevRef"=w425:T8)  [unwired: 2 in, 6 out]
            n129 = call <vilib>:"CTRE_Phoenix_MotorControl_Set.vi"("Output"=0.0, "Control Mode"=w420, "PhoenixMotorControlDevRef"=w414) -> ("PhoenixMotorControlDevRef"=w410:T3)  [unwired: 7 in, 1 out]
            n130 = call-poly <vilib>:"NT Write Value.vi"("Numeric Array"=w431, "Name"="RobotDrive Motors") -> ()  [unwired: 9 in, 1 out]
            n131 = call <vilib>:"WPI_MotorControlSetOutput.vi"("Output"=w422, "MotorControlDevRef"=w415) -> ("MotorControlDevRef"=w411:T3)  [unwired: 7 in, 2 out]
            n132 = call <vilib>:"WPI_MotorControlSetOutput.vi"("Output"=w422, "MotorControlDevRef"=w416) -> ("MotorControlDevRef"=w412:T3)  [unwired: 7 in, 2 out]
          }
        }
        frame #5 {
          n133 = Tick Count (ms)() -> (millisecond timer value=w432:u32)
          n134 = while {
            tunnel: w432 -> [w455]
            tunnel: 5000 -> [w454]
            tunnel: [w451] -> _
            tunnel: [w449] -> _
            tunnel: w437 -> [w450]
            tunnel: w439 -> [w445]
            tunnel: w438 -> [w444]
            tunnel: w436 -> [w442]
            tunnel: w435 -> [w441]
            tunnel: w434 -> [w440]
            stop <- w453 stop-if-true
            w446 = T13 0 items=["PercentOutput"=0, "Position"=1, "Velocity"=2, "Current"=3, "Follower"=5, "MotionProfile"=6, "MotionMagic"=7, "MotionProfileArc"=10, "Disabled"=15] ("Control Mode")
            w443 = 0.0 ("Output")
            w448 = 0.0 ("Output")
            # "Index"
            # "Flywheel"
            # "Stop all"
            n135 = call <vilib>:"WPI_MotorControlSetOutput.vi"("Output"=w443, "MotorControlDevRef"=w450) -> ("MotorControlDevRef"=w449:T3)  [unwired: 7 in, 2 out]
            n136 = call "Timeout.vi"("Start Time In"=w455, "Limit In"=w454) -> ("Timeout"=w453:bool)  [unwired: 8 in, 1 out]
            n137 = call <vilib>:"WPI_MotorControlSetOutput.vi"("Output"=w443, "MotorControlDevRef"=w444) -> ()  [unwired: 7 in, 3 out]
            n138 = call <vilib>:"WPI_RobotDriveArcadeDrive_Standard(NoSaturation).vi"("Y axis value"=0.0, "RobotDriveDevRef"=w445) -> ("Motor Values"=w457:dbl[], "RobotDriveDevRef"=w451:T8)  [unwired: 2 in, 6 out]
            n139 = call <vilib>:"CTRE_Phoenix_MotorControl_Set.vi"("Output"=0.0, "Control Mode"=w446, "PhoenixMotorControlDevRef"=w440) -> ()  [unwired: 7 in, 2 out]
            n140 = call-poly <vilib>:"NT Write Value.vi"("Numeric Array"=w457, "Name"="RobotDrive Motors") -> ()  [unwired: 9 in, 1 out]
            n141 = call <vilib>:"WPI_MotorControlSetOutput.vi"("Output"=w448, "MotorControlDevRef"=w441) -> ()  [unwired: 7 in, 3 out]
            n142 = call <vilib>:"WPI_MotorControlSetOutput.vi"("Output"=w448, "MotorControlDevRef"=w442) -> ()  [unwired: 7 in, 3 out]
          }
        }
      }
    }
  }
